vi "myRIO_BRig_RT_dataExp_runTime_seconds.vi"() -> (2 "output_RunTime_minutes":i32)   [LabVIEW 2014]
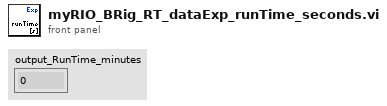
[diagram p1: front panel]
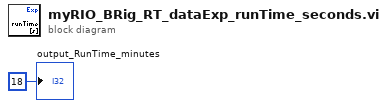
[diagram p0: block diagram]
diagram:
  "output_RunTime_minutes" <- 18 ("output_iBlock")
